vi "Read StateManager.vi"(8 "error in (no error)":errorcluster, 11 "ICS in":refnum<class "ICS.lvclass">) -> (0 "error out":errorcluster, 2 "StateManager":refnum<class "StateManager.lvclass">, 3 "ICS out":refnum<class "ICS.lvclass">, 4 "in motion":bool)   [LabVIEW 2018, in "ICS.lvclass"]
uses:
  ICS.lvclass
  StateManager/StateManager.lvclass
  ICS.lvclass/ICS.ctl
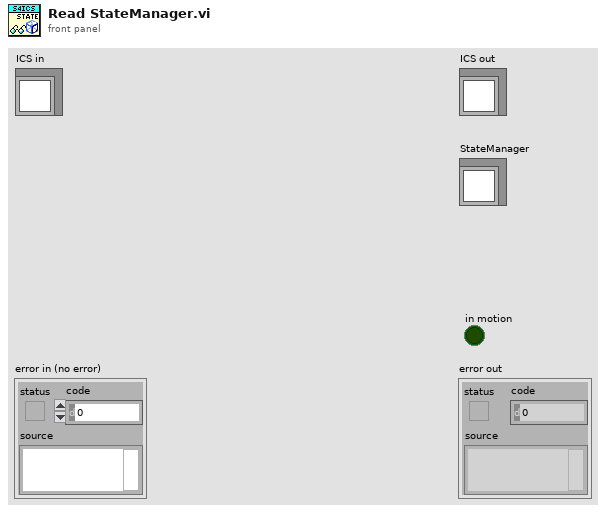
[diagram p1: front panel]
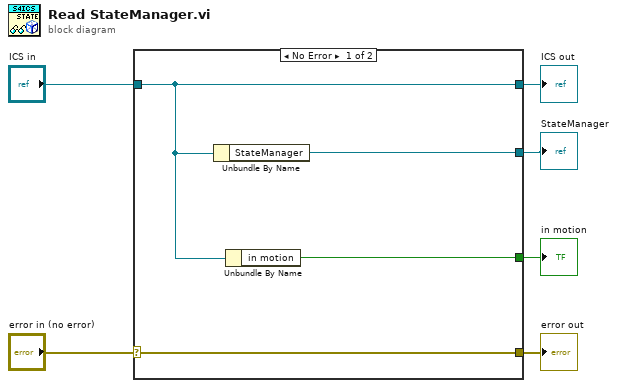
[diagram p0: block diagram]
diagram:
  n1 = case shown="No Error" "error in (no error)" {
    selector: "error in (no error)" -> [w10 w11]
    tunnel: [w10 w11] -> w5
    tunnel: [w8 w12] -> w3
    tunnel: "ICS in" -> [w8 w12]
    tunnel: [w9 _] -> w2
    tunnel: [w7 _] -> w1
    frame No Error {
      n2 = Unbundle By Name(w8) -> ("StateManager"=w9:refnum<class "StateManager.lvclass">)
      n3 = Unbundle By Name(w8) -> ("in motion"=w7:bool)
    }
    frame Error {
    }
  }
  "error out" <- w5
  "ICS out" <- w3
  "StateManager" <- w2
  "in motion" <- w1
